vi "Teleop.vi"(10 "Match Info":T2={"Autonomous Elapsed Seconds"=0.0, "TeleOp Elapsed Seconds"=0.0, "Disabled Elapsed Seconds"=0.0, "Visited Autonomous"=FALSE, "Visited TeleOp"=FALSE, "Visited Disabled"=FALSE, "Autonomous Settings"={"Autonomous Style"=enum."Independent", "VI Refnum"=refnum}}, 11 "Call Context":T3) -> ()   [LabVIEW 2020]
doc: "This VI is called for each enabled TeleOp packet received from the DS. It is typically used to read from joysticks and other inputs and update I/O or setpoints for timed control loops. It should complete and return within 20 milliseconds or risk missing DS packets."
uses:
  <vilib>/Rock Robotics/WPI/DriverStation/WPI_DriverStationDerivedRobotMode.ctl
  <vilib>/Rock Robotics/WPI/DriverStation/WPI_DriverStationMatch Info.ctl
  <vilib>/Rock Robotics/WPI/Utilities/WPI_GetSetVariantRefNum.vi
  <vilib>/Rock Robotics/Network Tables/NT Write Numeric Array.vi
  <vilib>/Rock Robotics/Network Tables/NT Write Boolean Array.vi
  Framework/Robot Global Data.vi
panel:
  in  "Teleops":T1={"Drive"=TRUE, "Intake"=TRUE, "Climb"=TRUE, "Transfer"=TRUE, "Shooter"=TRUE}
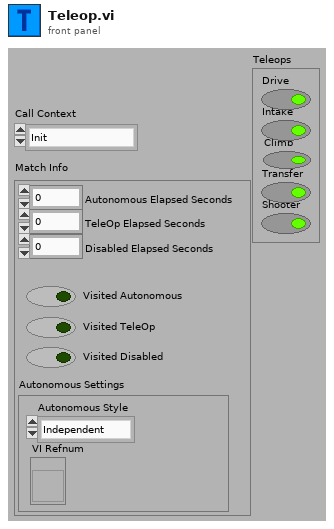
[diagram p1: front panel]
types:
  T1 = cluster{"Drive":bool, "Intake":bool, "Climb":bool, "Transfer":bool, "Shooter":bool}
  T2 = typedef "WPI_DriverStationMatch Info.ctl" = cluster{"Autonomous Elapsed Seconds":dbl, "TeleOp Elapsed Seconds":dbl, "Disabled Elapsed Seconds":dbl, "Visited Autonomous":bool, "Visited TeleOp":bool, "Visited Disabled":bool, "Autonomous Settings":cluster{"Autonomous Style":enum16{"Iterative", "Independent"}, "VI Refnum":refnum<vi>}}
  T3 = typedef "WPI_DriverStationDerivedRobotMode.ctl" = enum16{"Init", "Execute", "Stop"}
  T4 = typedef "numlock.ctl" = cluster{"tdms file out":refnum<k34>, "Default log level (info)":enum16{"trace", "debug", "info", "warn", "error"}}
  T5 = typedef "WPI_JoystickDevRef.ctl" = cluster{"Device":T6}
  T6 = typedef "WPI_JoystickDeviceEnum.ctl" = enum16{"USB 0", "USB 1", "USB 2", "USB 3", "USB 4", "USB 5"}
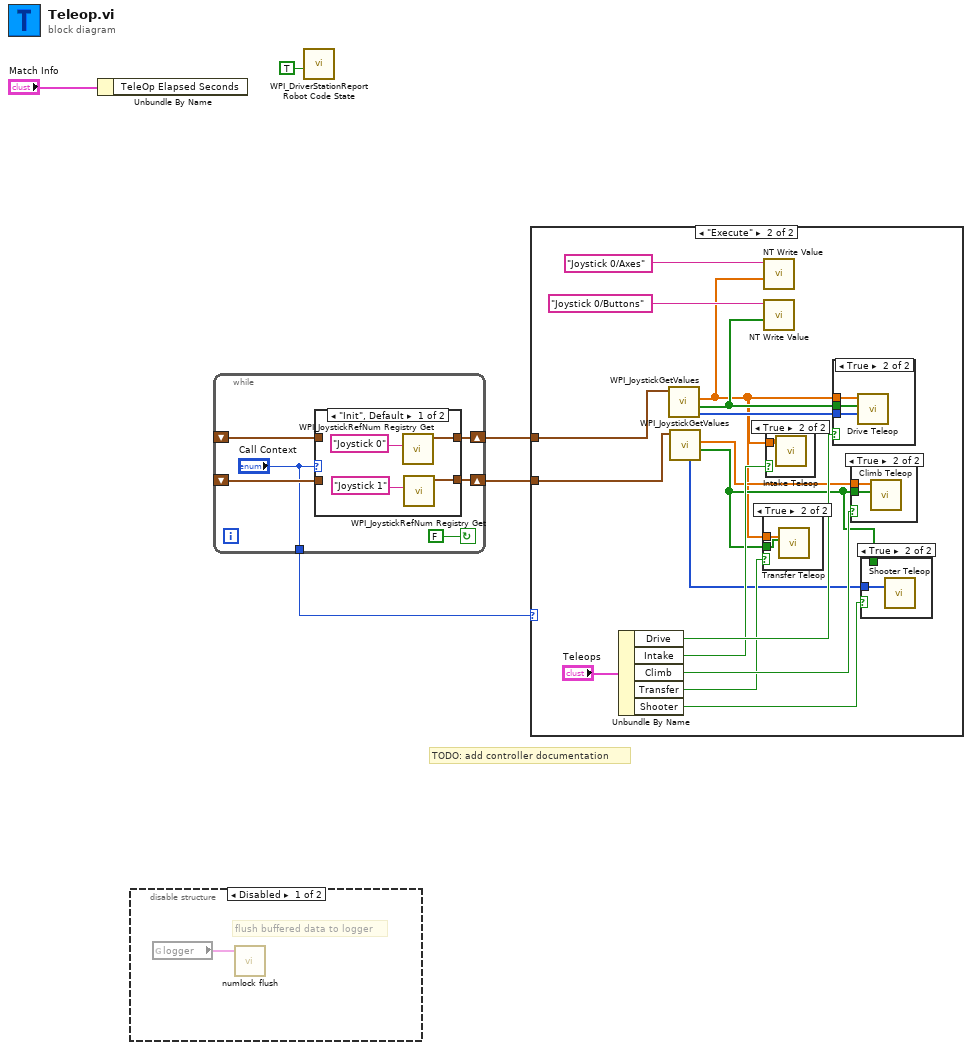
[diagram p0: block diagram]
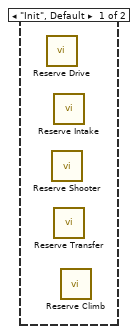
[diagram p2: hidden frame]
diagram:
  # "TODO: add controller documentation"
  n1 = Unbundle By Name("Match Info") -> ()  [unwired: 1 out]
  n2 = disable-structure shown="Disabled" {
    frame Disabled {
      # "flush buffered data to logger"
      n3 = global read "Robot Global Data.vi" "logger"() -> (w6:T4)
      n4 = call "numlock flush.vi"("logger"=w6) -> ()  [unwired: 9 in, 2 out]
    }
    frame Enabled {
    }
  }
  n5 = while {
    shift-right: [w12] -> w3
    shift-left: _ -> [w11]
    shift-right: [w9] -> w2
    shift-left: _ -> [w8]
    tunnel: ["Call Context"] -> w1
    stop <- FALSE continue-if-true
    n6 = case shown="\"Init\", Default" "Call Context" {
      tunnel: [w15 w18] -> w12
      tunnel: w11 -> [_ w18]
      tunnel: [w13 w17] -> w9
      tunnel: w8 -> [_ w17]
      frame "Init", Default {
        n7 = call <vilib>:"WPI_JoystickRefNum Registry Get.vi"("refnum name"="Joystick 0") -> ("JoystickDevRef"=w15:T5)  [unwired: 1 in, 9 out]
        n8 = call <vilib>:"WPI_JoystickRefNum Registry Get.vi"("refnum name"="Joystick 1") -> ("JoystickDevRef"=w13:T5)  [unwired: 1 in, 9 out]
      }
      frame "Execute" {
      }
    }
  }
  n9 = call <vilib>:"WPI_DriverStationReport Robot Code State.vi"("TeleOp"=TRUE ("Autonomous")) -> ()  [unwired: 10 in, 1 out]
  n10 = case shown="\"Execute\"" w1 {
    tunnel: w3 -> [_ w34]
    tunnel: w2 -> [_ w29]
    frame "Init", Default {
      n11 = call "Reserve Drive.vi"() -> ()  [unwired: 11 in, 1 out]
      n12 = call "Reserve Shooter.vi"() -> ()  [unwired: 11 in, 1 out]
      n13 = call "Reserve Intake.vi"() -> ()  [unwired: 11 in, 1 out]
      n14 = call "Reserve Transfer.vi"() -> ()  [unwired: 11 in, 1 out]
      n15 = call "Reserve Climb.vi"() -> ()  [unwired: 11 in, 1 out]
    }
    frame "Execute" {
      n16 = Unbundle By Name("Teleops") -> ("Drive"=w27:bool, "Intake"=w26:bool, "Climb"=w25:bool, "Transfer"=w24:bool, "Shooter"=w23:bool)
      n17 = call <vilib>:"WPI_JoystickGetValues.vi"("JoystickDevRef"=w34) -> ("Buttons"=w30:bool[], "Axes"=w19:dbl[], "POVs"=w31:i16[])  [unwired: 6 in, 2 out]
      n18 = call <vilib>:"WPI_JoystickGetValues.vi"("JoystickDevRef"=w29) -> ("Buttons"=w21:bool[], "Axes"=w20:dbl[], "POVs"=w22:i16[])  [unwired: 6 in, 2 out]
      n19 = case shown="True" w24 {
        tunnel: w19 -> [_ w37]
        tunnel: w21 -> [_ w36]
        frame False {
        }
        frame True {
          n20 = call "Transfer Teleop.vi"("Buttons"=w36, "Axes"=w37) -> ()  [unwired: 10 in]
        }
      }
      n21 = call-poly <vilib>:"NT Write Value.vi"("Numeric Array"=w19, "Name"="Joystick 0/Axes") -> ()  [unwired: 9 in, 1 out]
      n22 = call-poly <vilib>:"NT Write Value.vi"("Boolean Array"=w30, "Name"="Joystick 0/Buttons") -> ()  [unwired: 9 in, 1 out]
      n23 = case shown="True" w26 {
        tunnel: w19 -> [_ w40]
        frame False {
        }
        frame True {
          n24 = call "Intake Teleop.vi"("Axes"=w40) -> ()  [unwired: 11 in]
        }
      }
      n25 = case shown="True" w27 {
        tunnel: w31 -> [_ w43]
        tunnel: w30 -> [_ w42]
        tunnel: w19 -> [_ w41]
        frame False {
        }
        frame True {
          n26 = call "Drive Teleop.vi"("POVs"=w43, "Boolean Array"=w42, "Axes"=w41) -> ()  [unwired: 9 in]
        }
      }
      n27 = case shown="True" w25 {
        tunnel: w21 -> [_ w39]
        tunnel: w20 -> [_ w38]
        frame False {
        }
        frame True {
          n28 = call "Climb Teleop.vi"("Buttons"=w39, "Axes"=w38) -> ()  [unwired: 10 in]
        }
      }
      n29 = case shown="True" w23 {
        tunnel: w22 -> [_ w35]
        tunnel: w21 -> [_ _]
        frame False {
        }
        frame True {
          n30 = call "Shooter Teleop.vi"("POVs"=w35) -> ()  [unwired: 11 in]
        }
      }
    }
  }
